vi "proc_command.vi"(5 "recieve interval [ms]":i32=100, 7 "timeout [ms]":i32=1000, 8 "error in":errorcluster, 9 "read buffer size":i32, 10 "write buffer":string, 11 "process instance handle in":u32[](array[numeric])) -> (0 "error out":errorcluster, 1 "bytes read":i32, 2 "read buffer":string, 3 "process instance handle out":u32[](array[numeric]), 4 "exited":bool)   [LabVIEW 2011]
doc: "Flushes data in process stdout pipe, sends write buffer to stdin pipe, stores response from stdout pipe to read buffer. Reading from stdout implements two timeouts: first byte timeout and maximum chunk receive interval. VI defaultly waits 1s for first response byte and stops receiving if interval between bytes exeeds 100ms."
panel:
  in  "exit mem":i32
  in  "read mem":i32
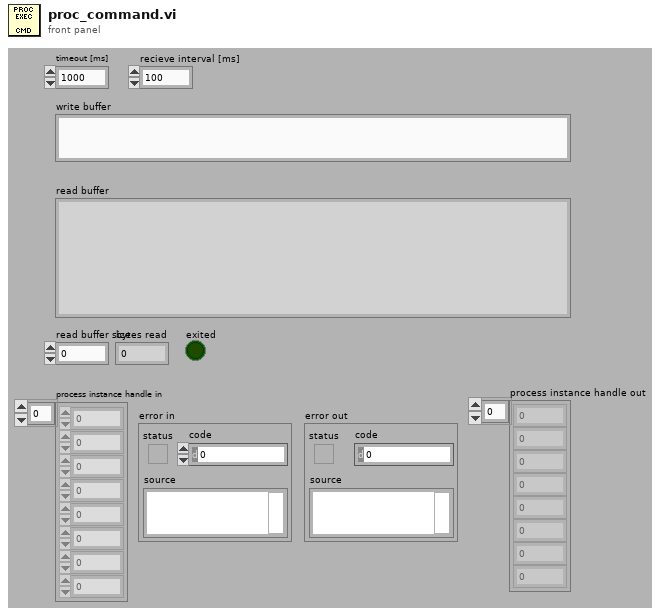
[diagram p1: front panel]
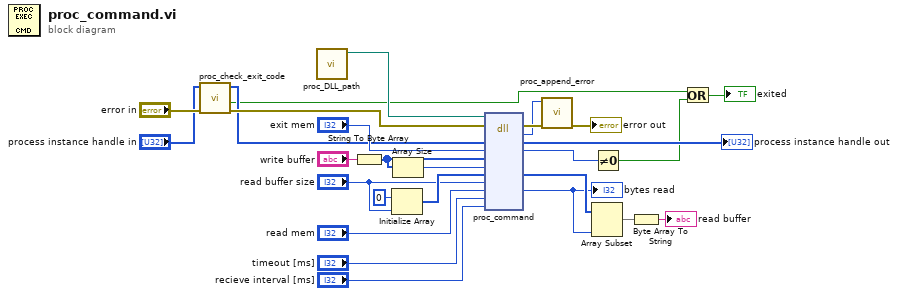
[diagram p0: block diagram]
diagram:
  n1 = call "proc_check_exit_code.vi"("error in"="error in", "instance handle in"="process instance handle in") -> ("error out"=w6:errorcluster, "exited"=w1:bool, "instance handle out"=w4:u32[])  [unwired: 5 in, 2 out]
  n2 = call "proc_DLL_path.vi"() -> ("path out"=w27:path)  [unwired: 10 in, 1 out]
  n3 = String To Byte Array(string="write buffer") -> (unsigned byte array=w21:u8[])
  n4 = Initialize Array(u8 0 ("element"), "read buffer size") -> (w19:u8[])
  n5 = Array Size(array=w21) -> (size(s)=w20:i32)
  n6 = dll-call lib="lv_proc.dll" fn="proc_command"(path in=w27, error in=w6, "proc"=w4, "exit"="exit mem", "command"=w21, "cmdlen"=w20, "buffer"=w19, "buflen"="read buffer size", "read"="read mem", "timeout"="timeout [ms]", "interval"="recieve interval [ms]") -> (error out=w12:errorcluster, "error"=w10:i32, "proc"=→"process instance handle out":u32[], "exit"=w8:i32, "buffer"=w16:u8[], "read"=w15:i32)  [unwired: 6 in, 1 out]
  "bytes read" <- w15
  n7 = call "proc_append_error.vi"("error in"=w12, "code in"=w10) -> ("error out"=→"error out":errorcluster)  [unwired: 8 in, 1 out]
  n8 = Array Subset(array=w16, length=w15) -> (w24:u8[])  [unwired: 1 in]
  n9 = Not Equal To 0?(x=w8) -> (x != 0?=w2:bool)
  n10 = Byte Array To String(unsigned byte array=w24) -> (string=→"read buffer":string)
  n11 = Or(x=w1, y=w2) -> (x .or. y?=→"exited":bool)
